vi "ADC_READ VHLTHx VLLTHx.vi"(0 "ftHandle_out 2":u32, 1 "Sumador":u8, 2 "referenciar":bool, 3 "ref DAC\nTH0,TH1,TH2":u16, 4 "ref DAC\nTH3,TH4,TH5":u16, 5 "error out 2":errorcluster, 8 "Espera acceso FT":u32) -> (13 "WRITE OK":bool, 14 "ftHandle_out":u32, 15 "HLTHx":dbl, 16 "LLTHx":dbl, 19 "error out":errorcluster)   [LabVIEW 2019]
uses:
  ASIC_Valores dac_mux_ena.ctl
  Global cuenta erroes.vi
  <vilib>/Analysis/NI_AALBase.lvlib
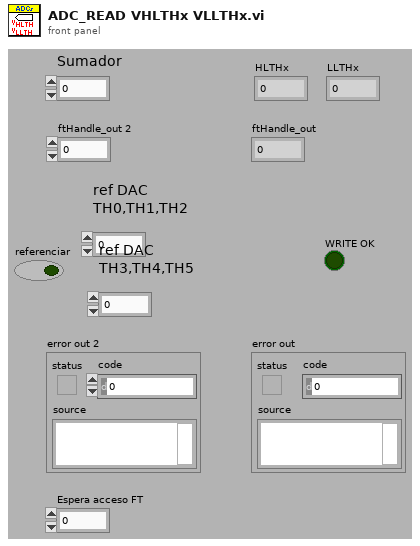
[diagram p1: front panel]
types:
  T1 = typedef "ASIC_Valores dac_mux_ena.ctl" = enum16{"---NULL 0--", "HLTH0 (ADD A)", "HLTH1 (ADD B)", "HLTH2 (ADD C)", "LLTH0 (ADD A)", "LLTH1 (ADD B)", "LLTH2 (ADD C)", "---NULL 1--"}
  T2 = typedef "global erroes cluster.ctl" = cluster{"Errores FPGA":i32, "Errores Asic":i32, "Errores ADC adq":i32, "Errores ADC Asic":i32}
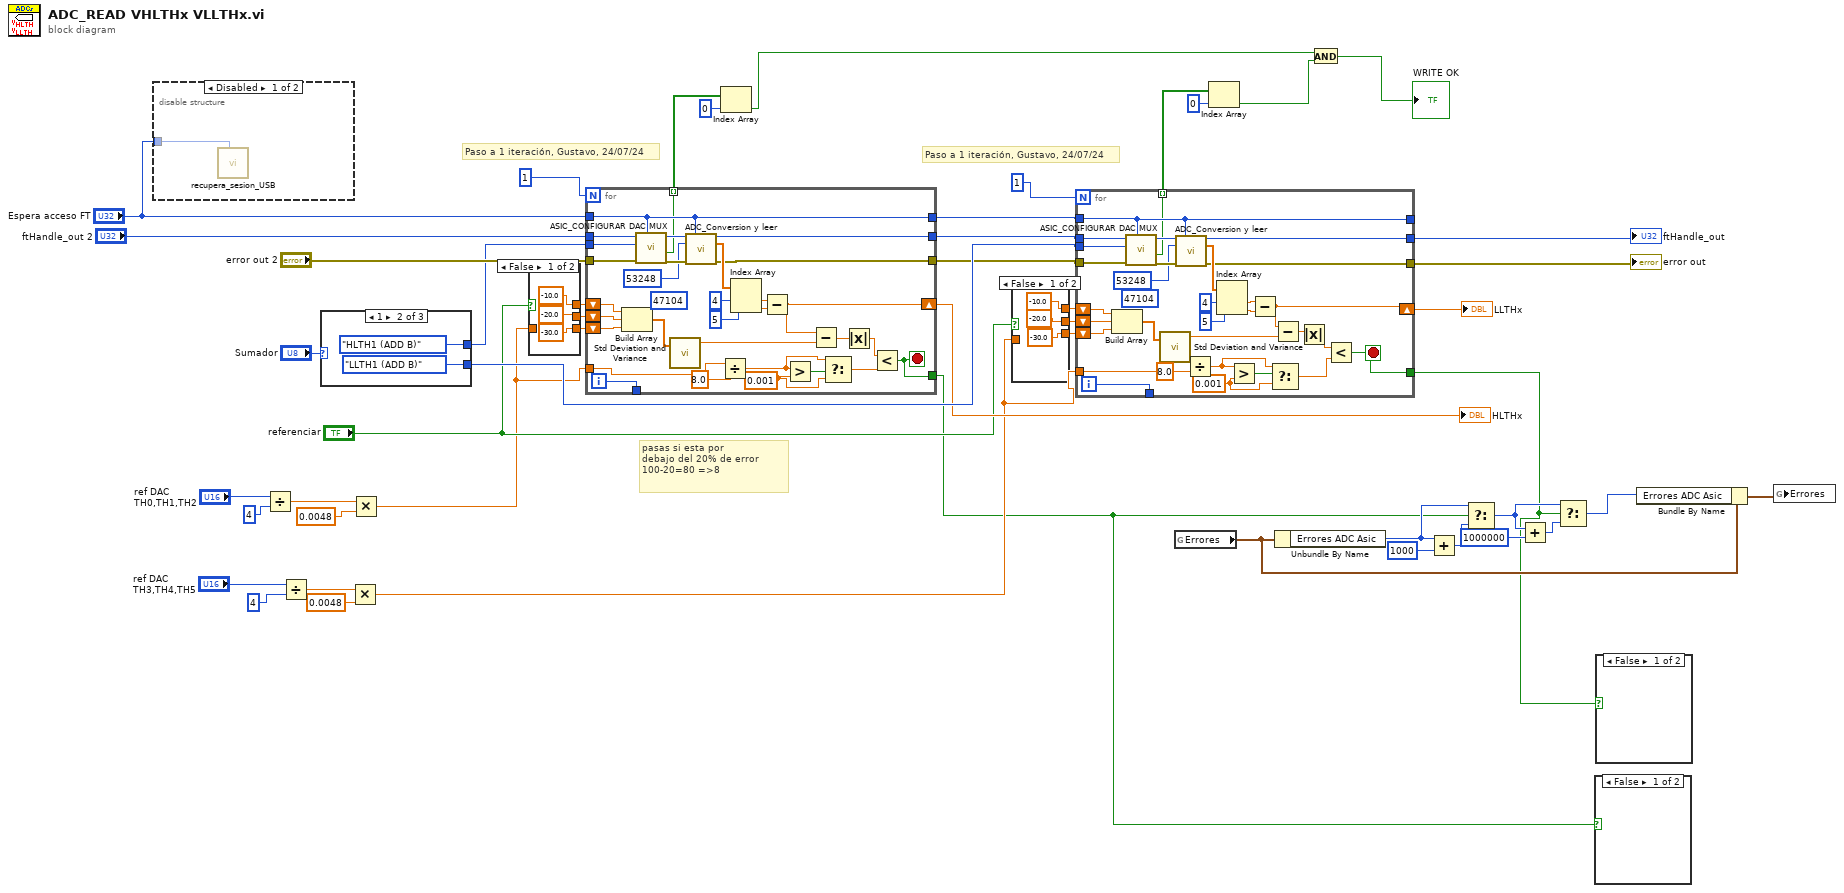
[diagram p0: block diagram]
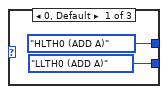
[diagram p7: hidden frame]
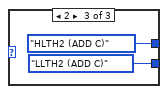
[diagram p8: hidden frame]
diagram:
  # "Paso a 1 iteración, Gustavo, 24/07/24"
  # "Paso a 1 iteración, Gustavo, 24/07/24"
  # "pasas si esta por \ndebajo del 20% de error\n100-20=80 =>8"
  n1 = disable-structure shown="Disabled" {
    disable-tunnel: "Espera acceso FT" -> [w51 _]
    frame Disabled {
      n2 = call "recupera_sesion_USB.vi"("Espera acceso USB"=w51) -> ()  [unwired: 9 in, 2 out]
    }
    frame Enabled {
    }
  }
  n3 = Divide(x="ref DAC\nTH0,TH1,TH2", y=u16 4) -> (x/y=w25:dbl)
  n4 = Divide(x="ref DAC\nTH3,TH4,TH5", y=u16 4) -> (x/y=w24:dbl)
  n5 = case shown="1" "Sumador" {
    tunnel: [ASIC_Valores_dac_mux_ena."HLTH0 (ADD A)" ("dac mux(0..7)") ASIC_Valores_dac_mux_ena."HLTH1 (ADD B)" ("dac mux(0..7)") ASIC_Valores_dac_mux_ena."HLTH2 (ADD C)" ("dac mux(0..7)")] -> w48
    tunnel: [ASIC_Valores_dac_mux_ena."LLTH0 (ADD A)" ("dac mux(0..7)") ASIC_Valores_dac_mux_ena."LLTH1 (ADD B)" ("dac mux(0..7)") ASIC_Valores_dac_mux_ena."LLTH2 (ADD C)" ("dac mux(0..7)")] -> w39
    frame 0, Default {
    }
    frame 1 {
    }
    frame 2 {
    }
  }
  n6 = Multiply(x=w24, y=0.0048) -> (x*y=w26:dbl)
  n7 = Multiply(x=w25, y=0.0048) -> (x*y=w27:dbl)
  n8 = case shown="False" "referenciar" {
    tunnel: [-10.0 w61] -> w47
    tunnel: [-20.0 w61] -> w46
    tunnel: [-30.0 w61] -> w45
    tunnel: w27 -> [_ w61]
    frame False {
    }
    frame True {
    }
  }
  n9 = for {
    N: 1 -> [_]
    tunnel: "error out 2" -> [w84]
    tunnel: "ftHandle_out 2" -> [w83]
    tunnel: "Espera acceso FT" -> [w75]
    tunnel: [w82] -> w40
    tunnel: [w81] -> w38
    tunnel: w48 -> [w80]
    shift-right: [w71] -> w37
    shift-left: w47 -> [w79]
    shift-left: w46 -> [w78]
    shift-left: w45 -> [w77]
    tunnel: [w75] -> w41
    tunnel: w27 -> [w70]
    tunnel: [w68] -> w11
    tunnel: [w67] -> _
    tunnel: [w62] -> w7 mode=indexing
    i -> [w67]
    stop <- w68 stop-if-true
    w64 = 0.001 ("y")
    (unwired) u16 47104
    n10 = Build Array(w79, w78, w77) -> (w76:dbl[])
    n11 = call "ASIC_CONFIGURAR DAC MUX.vi"("Espera acceso USB"=w75, "error in"=w84, "dac mux(0..7)"=w80, "ftHandle_in"=w83) -> ("error out"=w87:errorcluster, "Write OK"=w62:bool, "ftHandle_out"=w86:u32)  [unwired: 5 in]
    n12 = call <vilib>:"Std Deviation and Variance.vi"("X"=w76) -> ("mean"=w74:dbl)  [unwired: 1 in, 2 out]
    n13 = call "ADC_Conversion y leer.vi"("ftHandle_in 2"=w86, "Espera acceso USB"=w75, "Registro Conversion (0xD000)"=u16 53248, "error in 2"=w87) -> ("ftHandle_out"=w82:u32, "Datos Canal (V)"=w88:dbl[], "error out"=w81:errorcluster)  [unwired: 6 in, 3 out]
    n14 = Divide(x=w70, y=8.0) -> (x/y=w65:dbl)
    n15 = Index Array(array=w88, index #1=4 ("index"), index #2=5 ("index")) -> (element #1=w91:dbl, element #2=w92:dbl)
    n16 = Subtract(x=w91, y=w92) -> (x-y=w71:dbl)
    n17 = Greater?(x=w65, y=w64) -> (0:w66:bool)
    n18 = Subtract(x=w71, y=w74) -> (x-y=w73:dbl)
    n19 = Select(t=w65, s=w66, f=w64) -> (s? t:f=w63:dbl)
    n20 = Absolute Value(x=w73) -> (abs(x)=w72:dbl)
    n21 = Less?(x=w72, y=w63) -> (x < y?=w68:bool)
  }
  "HLTHx" <- w37
  n22 = Index Array(array=w7, index=0) -> (element=w3:bool)
  n23 = case shown="False" "referenciar" {
    tunnel: [-10.0 w96] -> w44
    tunnel: [-20.0 w96] -> w43
    tunnel: [-30.0 w96] -> w42
    tunnel: w26 -> [_ w96]
    frame False {
    }
    frame True {
    }
  }
  n24 = for {
    N: 1 -> [_]
    tunnel: w38 -> [w119]
    tunnel: w40 -> [w118]
    tunnel: w41 -> [w98]
    tunnel: [w117] -> w10
    tunnel: [w116] -> w35
    tunnel: w39 -> [w115]
    shift-right: [w107] -> w36
    shift-left: w44 -> [w114]
    shift-left: w43 -> [w113]
    shift-left: w42 -> [w112]
    tunnel: [w98] -> _
    tunnel: w26 -> [w106]
    tunnel: [w104] -> w12
    tunnel: [w103] -> _
    tunnel: [w97] -> w4 mode=indexing
    i -> [w103]
    stop <- w104 stop-if-true
    w100 = 0.001 ("y")
    (unwired) u16 47104
    n25 = Build Array(w114, w113, w112) -> (w111:dbl[])
    n26 = call "ASIC_CONFIGURAR DAC MUX.vi"("Espera acceso USB"=w98, "error in"=w119, "dac mux(0..7)"=w115, "ftHandle_in"=w118) -> ("error out"=w122:errorcluster, "Write OK"=w97:bool, "ftHandle_out"=w121:u32)  [unwired: 5 in]
    n27 = call <vilib>:"Std Deviation and Variance.vi"("X"=w111) -> ("mean"=w110:dbl)  [unwired: 1 in, 2 out]
    n28 = call "ADC_Conversion y leer.vi"("ftHandle_in 2"=w121, "Espera acceso USB"=w98, "Registro Conversion (0xD000)"=u16 53248, "error in 2"=w122) -> ("ftHandle_out"=w117:u32, "Datos Canal (V)"=w123:dbl[], "error out"=w116:errorcluster)  [unwired: 6 in, 3 out]
    n29 = Divide(x=w106, y=8.0) -> (x/y=w101:dbl)
    n30 = Index Array(array=w123, index #1=4 ("index"), index #2=5 ("index")) -> (element #1=w126:dbl, element #2=w127:dbl)
    n31 = Greater?(x=w101, y=w100) -> (0:w102:bool)
    n32 = Subtract(x=w126, y=w127) -> (x-y=w107:dbl)
    n33 = Select(t=w101, s=w102, f=w100) -> (s? t:f=w99:dbl)
    n34 = Subtract(x=w107, y=w110) -> (x-y=w109:dbl)
    n35 = Absolute Value(x=w109) -> (abs(x)=w108:dbl)
    n36 = Less?(x=w108, y=w99) -> (x < y?=w104:bool)
  }
  "error out" <- w35
  "ftHandle_out" <- w10
  "LLTHx" <- w36
  n37 = global read "Global cuenta erroes.vi" "Errores"() -> (w22:T2)
  n38 = Index Array(array=w4, index=0) -> (element=w2:bool)
  n39 = Unbundle By Name(w22) -> ("Errores ADC Asic"=w17:i32)
  n40 = And(x=w3, y=w2) -> (x .and. y?=→"WRITE OK":bool)
  n41 = Add(x=w17, y=1000) -> (x+y=w18:i32)
  n42 = Select(t=w17, s=w11, f=w18) -> (s? t:f=w14:i32)
  n43 = Add(x=w14, y=1000000) -> (x+y=w15:i32)
  n44 = Select(t=w14, s=w12, f=w15) -> (s? t:f=w21:i32)
  n45 = case shown="False" w11 {
    frame False {
    }
    frame True {
    }
  }
  n46 = case shown="False" w12 {
    frame False {
    }
    frame True {
    }
  }
  n47 = Bundle By Name(cluster=w22, "Errores ADC Asic"=w21) -> (w23:T2)
  n48 = global write "Global cuenta erroes.vi" "Errores"(w23) -> ()
